vi "Main.vi"(11 "Module Admin":refnum<class "Delacor_lib_QMH_Module Admin.lvclass">) -> ()   [LabVIEW 2020, in "Main.lvlib"]
doc: "This template is based off of the Queued Message Handler design pattern and the Queued Message Handler project template that ships with LabVIEW.\n\nThe main difference is that the queue is private to this module and communication between modules is performed via Broadcast and Request events.\n\nRequest events are wrapped in public API methods and are handled in the Event Handling Loop (EHL) of this VI. Any module can register for Broadcast events sent by this module. The EHL generates messages based on user interface actions.\n\nThe Message Handling Loop (MHL) processes messages generated by the EHL, or by other messages. The messages are string values, so new messages can be added easily to the Message Cases case structure in the MHL. Each message cluster can also provide an optional value for Message Data, which is a variant that can be converted to whatever message-specific data is required.\n_____\nBased on Delacor QMH Project Template 5.0.0.82."
uses:
  Main.lvlib
  <vilib>/Delacor/Delacor QMH/Libraries/Module Admin_class/Delacor_lib_QMH_Module Admin.lvclass
  Module Data--cluster.ctl
  <vilib>/Delacor/Delacor QMH/Libraries/Message Queue_class/Delacor_lib_QMH_Message Queue.lvclass/Delacor_lib_QMH_Message Queue.ctl
  <vilib>/event_ctls.llb/eventvkey.ctl
  Stop Argument--cluster.ctl
  <vilib>/Delacor/Delacor QMH/Libraries/Module Admin_class/Delacor_lib_QMH_Module Admin.lvclass/Delacor_lib_QMH_Module Admin.ctl
  <vilib>/event_ctls.llb/usereventprio.ctl
  <vilib>/Delacor/Delacor QMH/Libraries/Message Queue_class/Delacor_lib_QMH_Enqueue Message (Single).vi
  <vilib>/Delacor/Delacor QMH/Libraries/Module Admin_class/Delacor_lib_QMH_Get External Launch.vi
  <vilib>/Utility/error.llb/Error Cluster From Error Code.vi
  <vilib>/ErrorRing/Error Ring.xnode
  <vilib>/Delacor/Delacor QMH/Libraries/Message Queue_class/Delacor_lib_QMH_Message Queue.lvclass
  History/History.lvlib
  Fallas/Fallas.lvlib
  Pruebas/Pruebas.lvlib
  Graficas/Graficas.lvlib
panel:
  out "stop?":bool
  out "date/time string":string
  out "Enum Param":enum16{"None", "Corriente", "SOC", "Temp"}(ring)=enum."Temp"
  in  "Salir":bool
  in  "Historial":bool
  in  "Pruebas":bool
  in  "Fallas":bool
  in  "Pagina Principal":bool
  in  "OK SOC":bool
  in  "SOC de Batería":dbl min=0.0 max=340.0 step=10.0 format="%#_g %"
  out "Bus DC Encendido":bool
  in  "Ok Temperatura":bool
  in  "Temperatura de Batería":dbl min=0.0 max=340.0 step=10.0 format="%#_g °C"
  in  "Ok Propulsion":bool
  in  "Corriente de Propulsión":dbl min=0.0 max=340.0 step=10.0 format="%#_g A"
  in  "Modo Propulsion":bool
  in  "Conexion a Linea de Carga":bool
  in  "Encender Generador":bool
  out "error out":errorcluster
  out "Status":string
  # "Operación del Sistema"
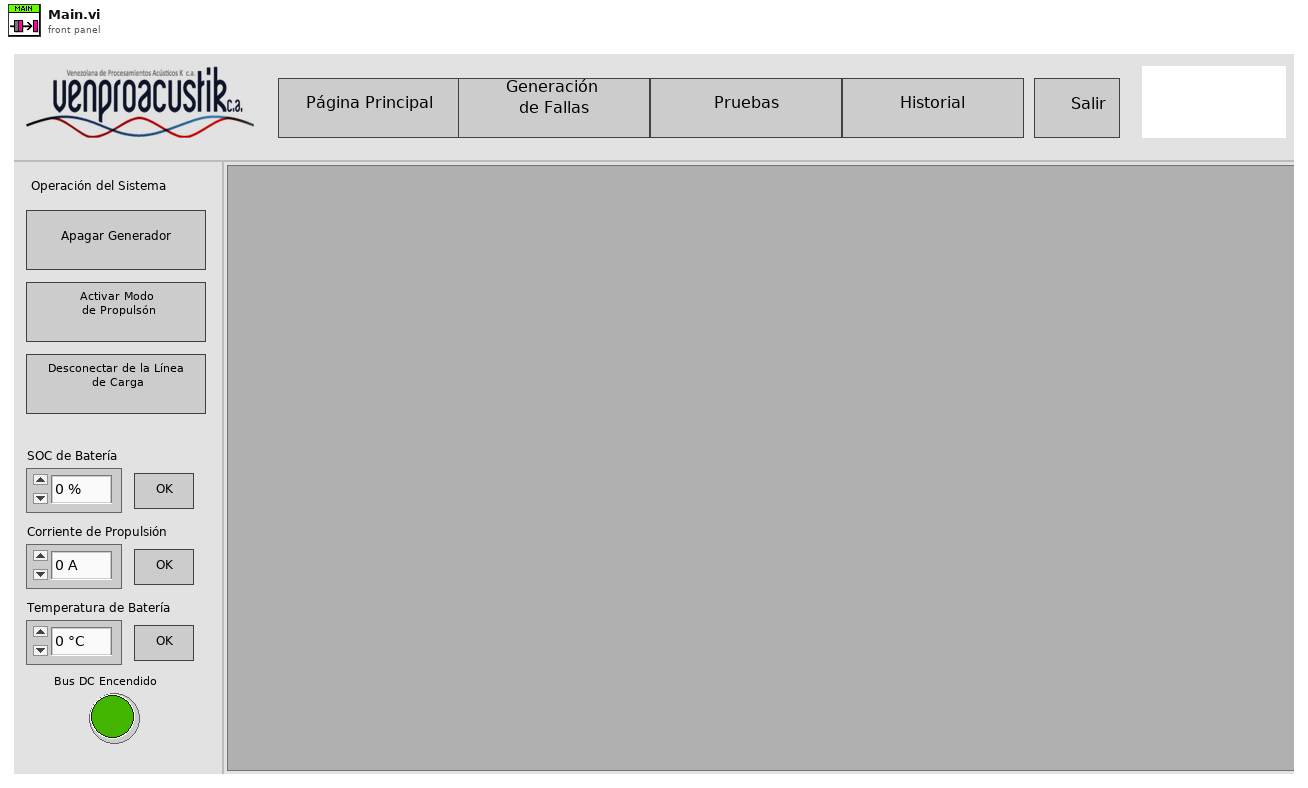
[diagram p1: front panel]
types:
  T1 = typedef "Main.lvlib/Request Events--cluster.ctl" = cluster{"Stop Module":refnum<user-event>, "Show Panel":refnum<user-event>, "Hide Panel":refnum<user-event>, "Get Module Execution Status":refnum<user-event>, "Show Diagram":refnum<user-event>}
  T2 = typedef "History.lvlib/Broadcast Events--cluster.ctl" = cluster{"Module Did Init":refnum<user-event>, "Status Updated":refnum<user-event>, "Error Reported":refnum<user-event>, "Module Did Stop":refnum<user-event>, "Update Module Execution Status":refnum<user-event>}
  T3 = typedef "Fallas.lvlib/Broadcast Events--cluster.ctl" = cluster{"Module Did Init":refnum<user-event>, "Status Updated":refnum<user-event>, "Error Reported":refnum<user-event>, "Module Did Stop":refnum<user-event>, "Update Module Execution Status":refnum<user-event>}
  T4 = typedef "Pruebas.lvlib/Broadcast Events--cluster.ctl" = cluster{"Module Did Init":refnum<user-event>, "Status Updated":refnum<user-event>, "Error Reported":refnum<user-event>, "Module Did Stop":refnum<user-event>, "Update Module Execution Status":refnum<user-event>, "Controles de relés de prueba actualizados":refnum<user-event>, "Valor de Medicion de Prueba Enviado":refnum<user-event>, "Valor de Modulacion Debugging Enviado":refnum<user-event>}
  T5 = typedef "Graficas.lvlib/Broadcast Events--cluster.ctl" = cluster{"Module Did Init":refnum<user-event>, "Status Updated":refnum<user-event>, "Error Reported":refnum<user-event>, "Module Did Stop":refnum<user-event>, "Update Module Execution Status":refnum<user-event>}
  T6 = typedef "Main.lvlib/Module Data--cluster.ctl" = cluster{"Status":string}
  T7 = typedef "eventvkey.ctl" = enum16{"ASCII", "Enter", "Return", "Shift", "Ctrl", "Alt", "Cmd", "Opt", "Caps", "NumLock", "Clear", "Break", "Up", "Down", "Left", "Right", "Insert", "Delete", "Home", "End", "PageUp", "PageDown", "Escape", "Help", "Pause", "ScrollLock", "F1", "F2", "F3", "F4", "F5", "F6", "F7", "F8", "F9", "F10", "F11", "F12", "F13", "F14", "F15", "F16", "F17", "F18", "F19", "F20", "F21", "F22", "F23", "F24", "Play", "VolumeUp", "VolumeDown", "Mute", "Two Byte Char"}
  T8 = typedef "Main.lvlib/Stop Argument--cluster.ctl" = cluster{"Origin":string, "Exit via Stop Module Req?":bool, "Wait for Module to stop?":bool}
  T9 = enum32{"invalid lock state", "Not Locked", "Locked (No Password)", "Password-protected"}
  T10 = typedef "usereventprio.ctl" = enum32{"high priority", "normal priority"}
  T11 = enum32{"Invalid", "Standard", "Closed", "Hidden", "Minimized", "Maximized"}
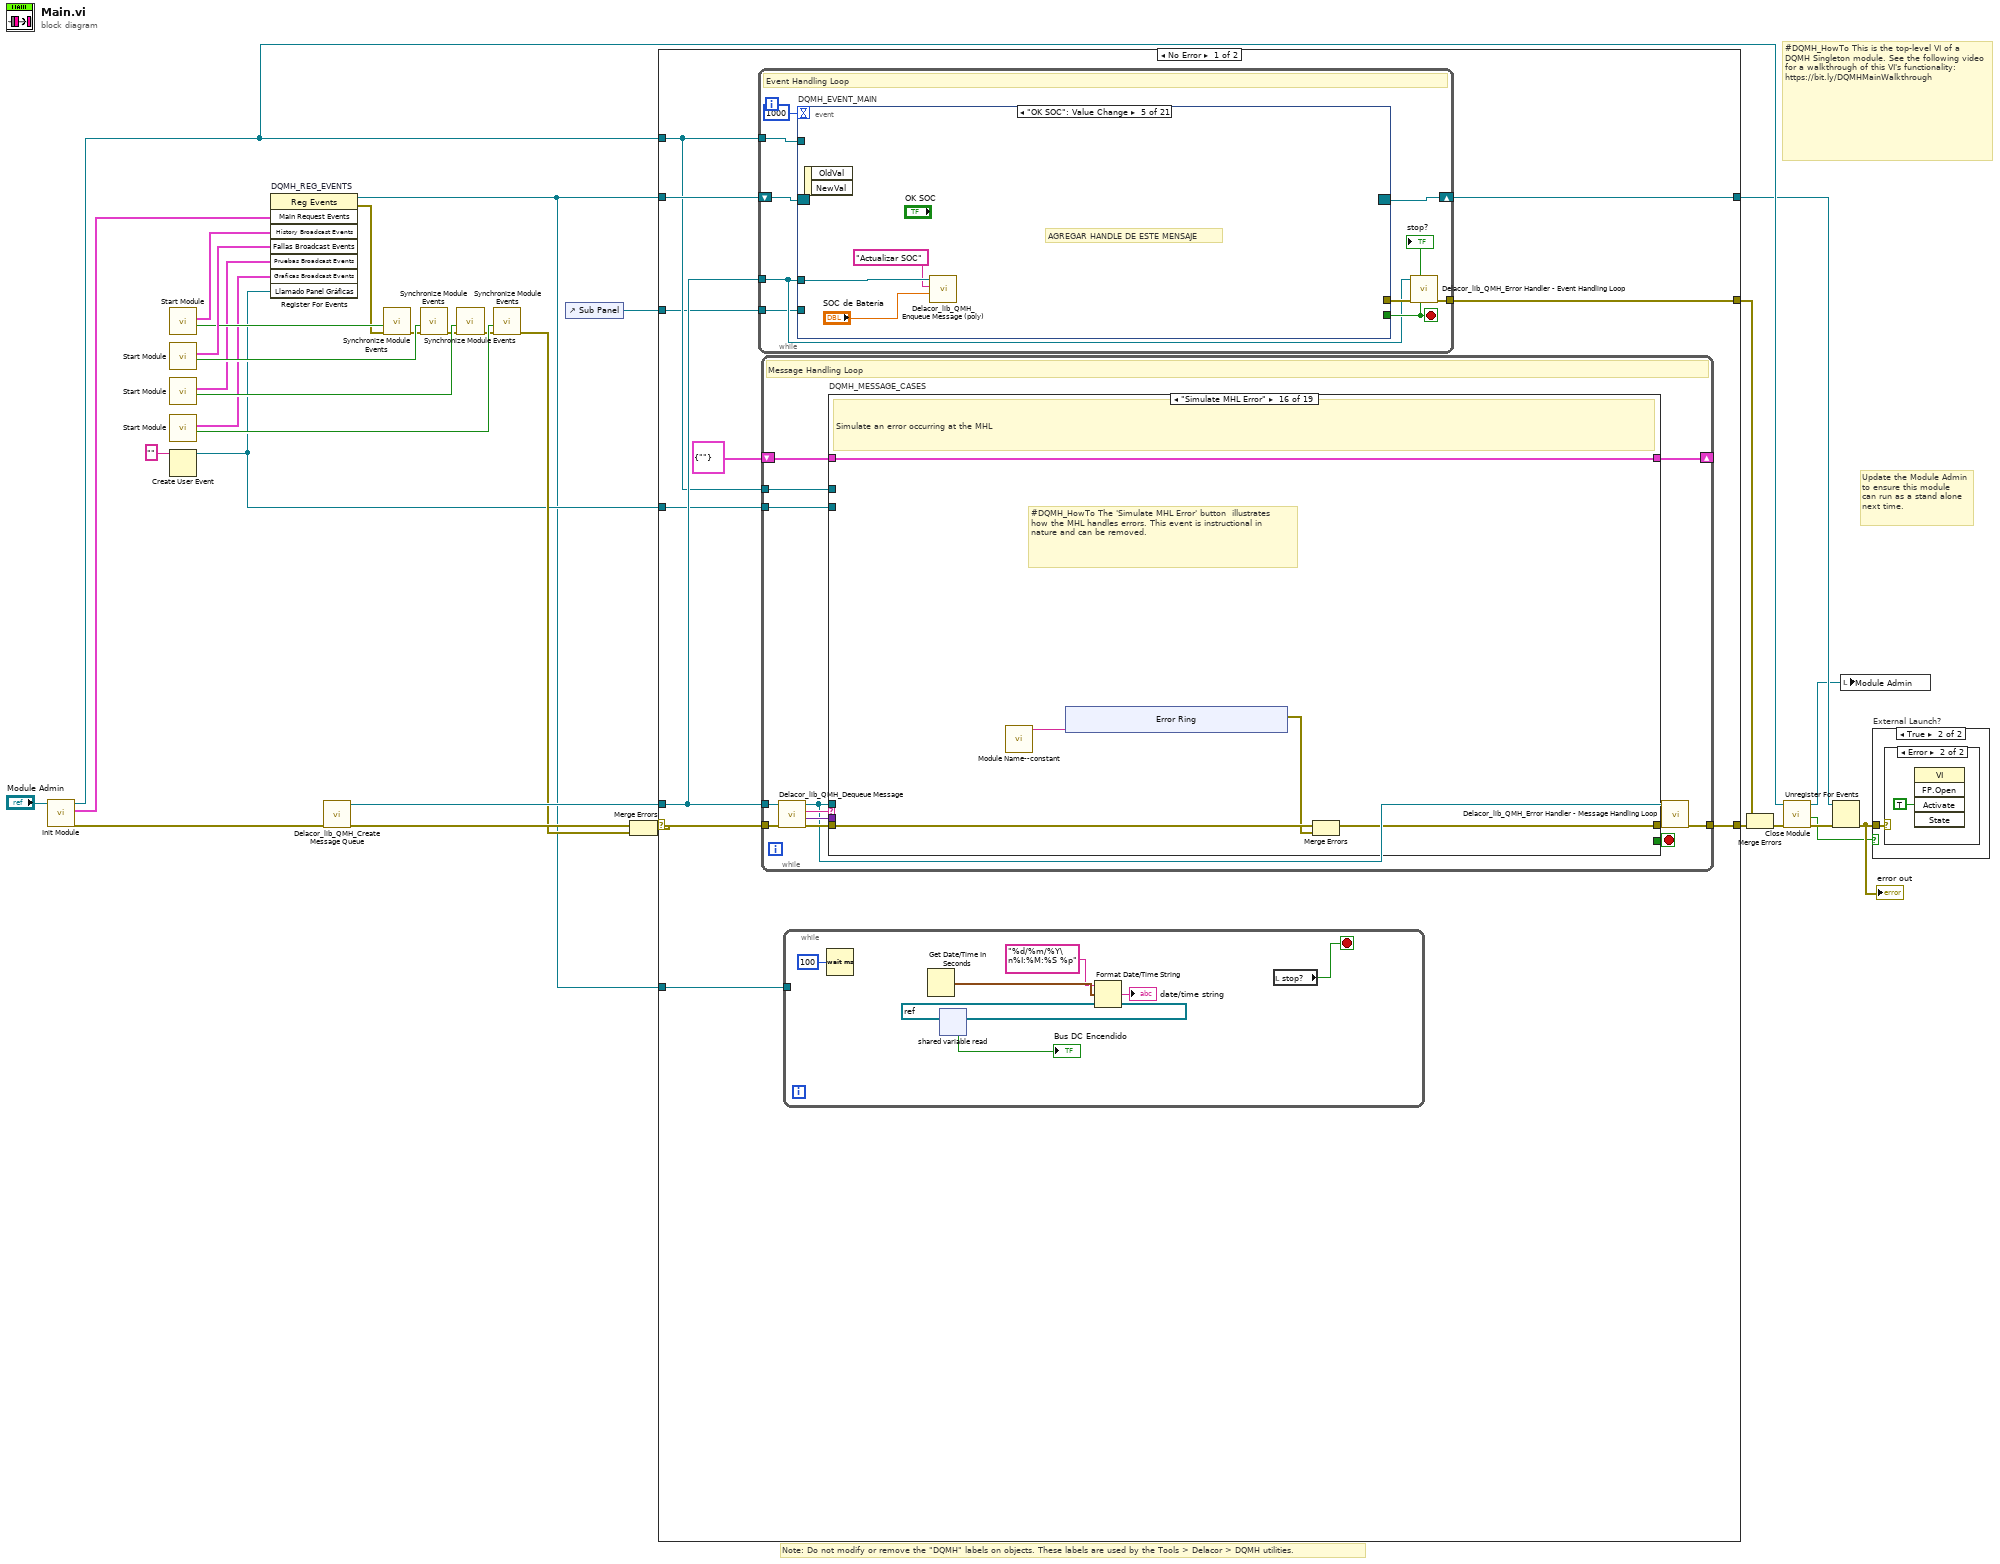
[diagram p0: block diagram]
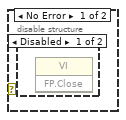
[diagram p3: hidden frame]
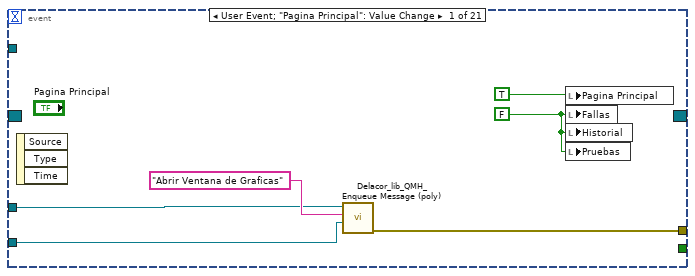
[diagram p5: hidden frame]
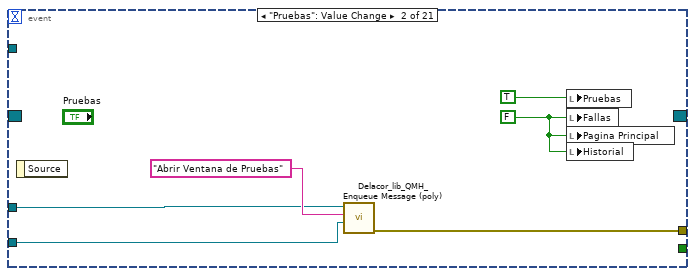
[diagram p6: hidden frame]
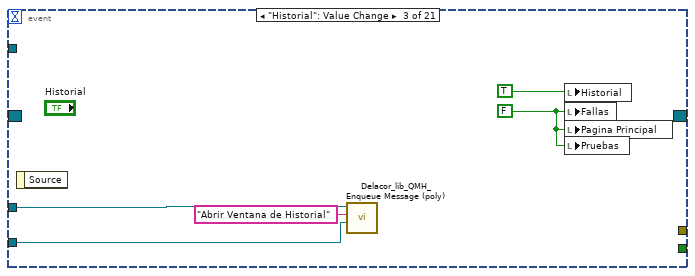
[diagram p7: hidden frame]
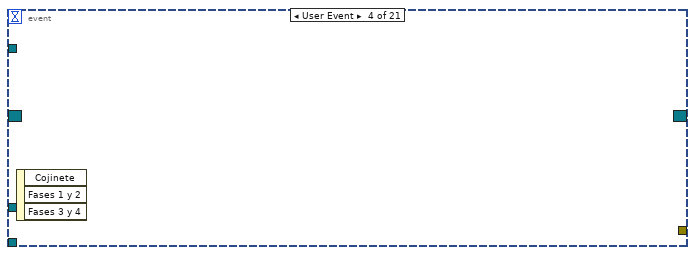
[diagram p8: hidden frame]
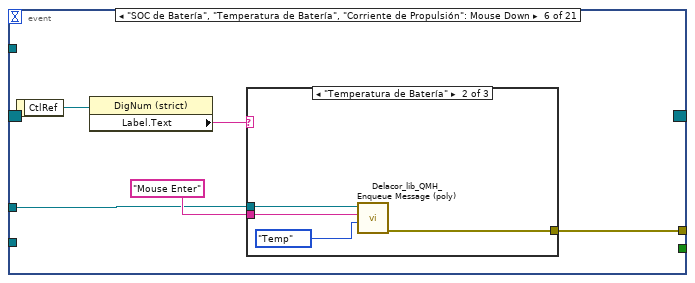
[diagram p9: hidden frame]
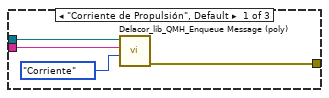
[diagram p10: hidden frame]
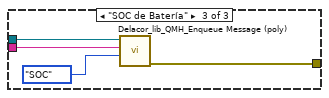
[diagram p11: hidden frame]
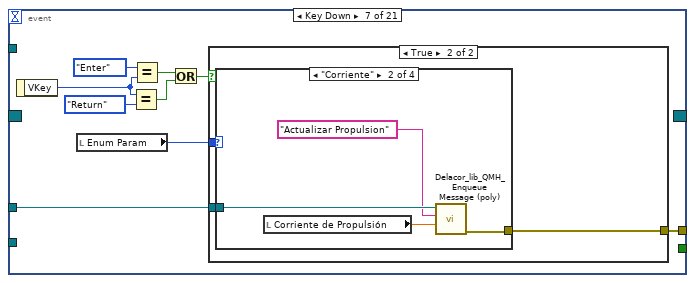
[diagram p12: hidden frame]
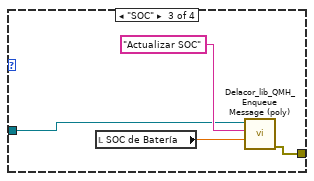
[diagram p15: hidden frame]
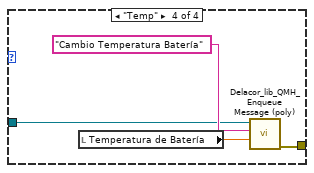
[diagram p16: hidden frame]
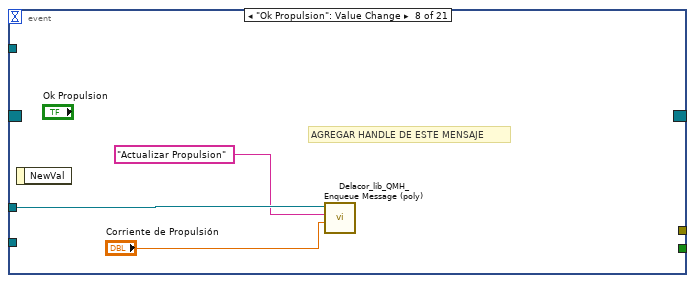
[diagram p17: hidden frame]
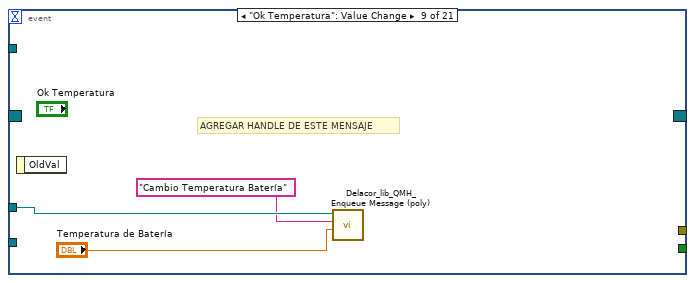
[diagram p18: hidden frame]
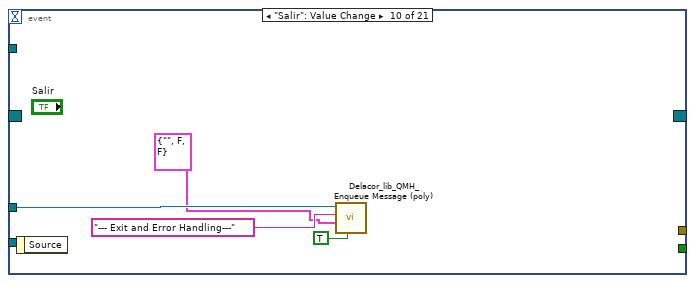
[diagram p19: hidden frame]
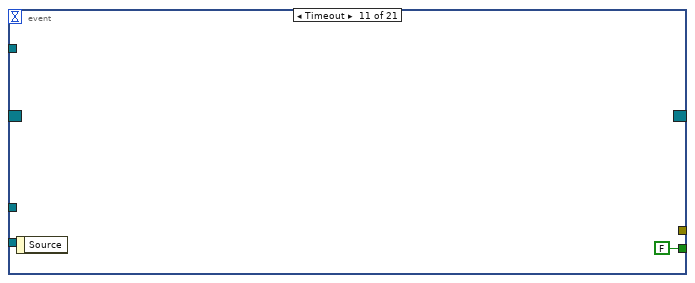
[diagram p20: hidden frame]
diagram:
  # "#DQMH_HowTo This is the top-level VI of a DQMH Singleton module. See the following video for a walkthrough of this VI's functionality: https://bit.ly/DQMHMainWalkthrough"
  # "Note: Do not modify or remove the \"DQMH\" labels on objects. These labels are used by the Tools > Delacor > DQMH utilities."
  # "Update the Module Admin to ensure this module can run as a stand alone next time."
  n1 = call "Init Module.vi"("Singleton Module Admin in"="Module Admin") -> ("error out"=w31:errorcluster, "Main Request Events"=w22:T1, "Singleton Module Admin out"=w24:refnum<class "Delacor_lib_QMH_Module Admin.lvclass">)  [unwired: 8 in]
  n2 = call "Start Module.vi"() -> ("Wait for Event Sync?"=w15:bool, "History Broadcast Events"=w17:T2)  [unwired: 8 in, 2 out]
  n3 = call "Start Module.vi"() -> ("Wait for Event Sync?"=w14:bool, "Fallas Broadcast Events"=w16:T3)  [unwired: 7 in, 3 out]
  n4 = call "Start Module.vi"() -> ("Wait for Event Sync?"=w11:bool, "Pruebas Broadcast Events"=w12:T4)  [unwired: 8 in, 2 out]
  n5 = call "Start Module.vi"() -> ("Wait for Event Sync?"=w9:bool, "Graficas Broadcast Events"=w10:T5)  [unwired: 8 in, 2 out]
  n6 = Create User Event(user event datatype="" ("Llamado Panel Gráficas")) -> (user event=w2:refnum<user-event>)  [unwired: 1 in, 1 out]
  n7 = register-events "DQMH_REG_EVENTS"(w22, w17, w16, w12, w10, w2) -> (reference out=w1:refnum<event-registration>, error out=w8:errorcluster)  [unwired: 2 in]
  n8 = call <vilib>:"Delacor_lib_QMH_Create Message Queue.vi"("error in (no error)"=w31) -> ("error out"=w26:errorcluster, "Message Queue"=w21:refnum<class "Delacor_lib_QMH_Message Queue.lvclass">)  [unwired: 9 in]
  n9 = call "Synchronize Module Events.vi"("error in (no error)"=w8, "Wait for Event Sync?"=w15) -> ("error out"=w7:errorcluster)  [unwired: 9 in]
  n10 = call "Synchronize Module Events.vi"("error in (no error)"=w7, "Wait for Event Sync?"=w14) -> ("error out"=w6:errorcluster)  [unwired: 9 in]
  n11 = call "Synchronize Module Events.vi"("error in (no error)"=w6, "Wait for Event Sync?"=w11) -> ("error out"=w5:errorcluster)  [unwired: 9 in]
  n12 = call "Synchronize Module Events.vi"("error in (no error)"=w5, "Wait for Event Sync?"=w9) -> ("error out"=w4:errorcluster)  [unwired: 9 in]
  n13 = control-ref of="Sub Panel"() -> (w13:refnum<vi>)
  n14 = Merge Errors(w26, w4) -> (w25:errorcluster)
  n15 = case shown="No Error" w25 {
    selector: w25 -> [w41 w408]
    tunnel: [w43 w407] -> w32
    tunnel: [w40 w413] -> w23
    tunnel: w1 -> [w38 w413]
    tunnel: w21 -> [w37 w406]
    tunnel: [w42 _] -> w29
    tunnel: w24 -> [w36 w409]
    tunnel: w13 -> [w35 _]
    tunnel: w2 -> [w34 _]
    tunnel: w1 -> [w33 _]
    frame No Error {
      n16 = while {
        tunnel: w37 -> [w53]
        shift-right: [w56] -> w40
        shift-left: w38 -> [w57]
        tunnel: [w58] -> w42
        tunnel: w36 -> [w54]
        tunnel: w35 -> [w52]
        stop <- w55 stop-if-true
        # "Event Handling Loop"
        n17 = event "DQMH_EVENT_MAIN" shown="[4] \"OK SOC\": Value Change" {
          selector: w57 -> [_ _ _ _ _ _ _ _ _ _ _ _ _ _ _ _ _ _ _ _ _]
          dyn-events: [_ _ _ _ _ _ _ _ _ _ _ _ _ _ _ _ _ _ _ _ _] -> w56
          timeout: 1000 -> [_ _ _ _ _ _ _ _ _ _ _ _ _ _ _ _ _ _ _ _ _]
          tunnel: [_ _ _ _ _ _ _ _ _ _ FALSE ("Discard?") _ _ _ _ _ TRUE ("Discard?") _ _ _ _] -> w55
          tunnel: w53 -> [w62 w66 w76 _ w79 w80 w98 w123 w126 w129 _ w136 _ _ _ _ w160 w168 w171 w175 w179]
          tunnel: [w61 w67 _ _ _ w82 w97 _ _ _ _ w132 _ _ w143 _ w163 w165 w170 w174 w181] -> w59
          tunnel: w54 -> [_ _ _ _ _ _ _ _ _ _ _ _ _ _ _ _ _ _ _ _ w178]
          tunnel: w52 -> [w60 w68 w72 _ _ _ _ _ _ _ _ w133 _ _ _ _ _ _ _ _ _]
          event User Event; "Pagina Principal": Value Change {
            w65 = FALSE ("Fallas")
            n18 = event-data() -> ()  [unwired: 1 in, 3 out]
            n19 = call-poly <vilib>:"Delacor_lib_QMH_Enqueue Message (poly).vi"("Message Data"=w60, "Message"="Abrir Ventana de Graficas", "Message Queue in"=w62) -> ("error out"=w61:errorcluster)  [unwired: 7 in, 1 out]
            n20 = local write "Pagina Principal"(TRUE ("Fallas")) -> ()
            n21 = local write "Fallas"(w65) -> ()
            n22 = local write "Historial"(w65) -> ()
            n23 = local write "Pruebas"(w65) -> ()
          }
          event "Pruebas": Value Change {
            w71 = FALSE ("Fallas")
            n24 = event-data() -> ()  [unwired: 1 in, 1 out]
            n25 = call-poly <vilib>:"Delacor_lib_QMH_Enqueue Message (poly).vi"("Message Data"=w68, "Message"="Abrir Ventana de Pruebas", "Message Queue in"=w66) -> ("error out"=w67:errorcluster)  [unwired: 7 in, 1 out]
            n26 = local write "Pruebas"(TRUE ("Fallas")) -> ()
            n27 = local write "Fallas"(w71) -> ()
            n28 = local write "Pagina Principal"(w71) -> ()
            n29 = local write "Historial"(w71) -> ()
          }
          event "Historial": Value Change {
            w74 = FALSE ("Fallas")
            n30 = event-data() -> ()  [unwired: 1 in, 1 out]
            n31 = call-poly <vilib>:"Delacor_lib_QMH_Enqueue Message (poly).vi"("Message Data"=w72, "Message"="Abrir Ventana de Historial", "Message Queue in"=w76) -> ()  [unwired: 7 in, 2 out]
            n32 = local write "Historial"(TRUE ("Fallas")) -> ()
            n33 = local write "Fallas"(w74) -> ()
            n34 = local write "Pagina Principal"(w74) -> ()
            n35 = local write "Pruebas"(w74) -> ()
          }
          event User Event {
            n36 = event-data() -> ()  [unwired: 1 in, 3 out]
          }
          event "OK SOC": Value Change {
            # "AGREGAR HANDLE DE ESTE MENSAJE"
            n37 = event-data() -> ()  [unwired: 1 in, 2 out]
            n38 = call-poly <vilib>:"Delacor_lib_QMH_Enqueue Message (poly).vi"("Message Data"="SOC de Batería", "Message"="Actualizar SOC", "Message Queue in"=w79) -> ()  [unwired: 7 in, 2 out]
          }
          event "SOC de Batería", "Temperatura de Batería", "Corriente de Propulsión": Mouse Down {
            n39 = event-data() -> ("CtlRef"=w84:refnum<vi>)  [unwired: 1 in]
            n40 = property class="DigNum (strict)"(reference=w84) -> ("Label.Text"=w83:string)  [unwired: 1 in, 2 out]
            n41 = case shown="\"Temperatura de Batería\"" w83 {
              tunnel: w80 -> [w88 w92 w96]
              tunnel: [w87 w91 w95] -> w82
              tunnel: "Mouse Enter" ("Message") -> [w85 w90 w93]
              frame "Corriente de Propulsión", Default {
                n42 = call-poly <vilib>:"Delacor_lib_QMH_Enqueue Message (poly).vi"("Message Data"=enum16{"None", "Corriente", "SOC", "Temp"}."Corriente", "Message"=w85, "Message Queue in"=w88) -> ("error out"=w87:errorcluster)  [unwired: 7 in, 1 out]
              }
              frame "Temperatura de Batería" {
                n43 = call-poly <vilib>:"Delacor_lib_QMH_Enqueue Message (poly).vi"("Message Data"=enum16{"None", "Corriente", "SOC", "Temp"}."Temp", "Message"=w90, "Message Queue in"=w92) -> ("error out"=w91:errorcluster)  [unwired: 7 in, 1 out]
              }
              frame "SOC de Batería" {
                n44 = call-poly <vilib>:"Delacor_lib_QMH_Enqueue Message (poly).vi"("Message Data"=enum16{"None", "Corriente", "SOC", "Temp"}."SOC", "Message"=w93, "Message Queue in"=w96) -> ("error out"=w95:errorcluster)  [unwired: 7 in, 1 out]
              }
            }
          }
          event Key Down {
            n45 = event-data() -> ("VKey"=w104:T7)  [unwired: 1 in]
            n46 = local read "Enum Param"() -> (w99:enum16{"None", "Corriente", "SOC", "Temp"})
            n47 = Equal?(x=w104, y=eventvkey."Return" ("VKey 2")) -> (x = y?=w101:bool)
            n48 = Equal?(x=eventvkey."Enter" ("VKey 2"), y=w104) -> (x = y?=w102:bool)
            n49 = Or(x=w102, y=w101) -> (x .or. y?=w100:bool)
            n50 = case shown="True" w100 {
              tunnel: w99 -> [_ w108]
              tunnel: w98 -> [_ w107]
              tunnel: [_ w106] -> w97
              frame False {
              }
              frame True {
                n51 = case shown="\"Corriente\"" w108 {
                  tunnel: w107 -> [_ w112 w114 w118]
                  tunnel: [_ w111 w113 w117] -> w106
                  frame "None", Default {
                  }
                  frame "Corriente" {
                    n52 = local read "Corriente de Propulsión"() -> (w109:dbl)
                    n53 = call-poly <vilib>:"Delacor_lib_QMH_Enqueue Message (poly).vi"("Message Data"=w109, "Message"="Actualizar Propulsion", "Message Queue in"=w112) -> ("error out"=w111:errorcluster)  [unwired: 7 in, 1 out]
                  }
                  frame "SOC" {
                    n54 = local read "SOC de Batería"() -> (w116:dbl)
                    n55 = call-poly <vilib>:"Delacor_lib_QMH_Enqueue Message (poly).vi"("Message Data"=w116, "Message"="Actualizar SOC", "Message Queue in"=w114) -> ("error out"=w113:errorcluster)  [unwired: 7 in, 1 out]
                  }
                  frame "Temp" {
                    n56 = local read "Temperatura de Batería"() -> (w120:dbl)
                    n57 = call-poly <vilib>:"Delacor_lib_QMH_Enqueue Message (poly).vi"("Message Data"=w120, "Message"="Cambio Temperatura Batería", "Message Queue in"=w118) -> ("error out"=w117:errorcluster)  [unwired: 7 in, 1 out]
                  }
                }
              }
            }
          }
          event "Ok Propulsion": Value Change {
            # "AGREGAR HANDLE DE ESTE MENSAJE"
            n58 = event-data() -> ()  [unwired: 1 in, 1 out]
            n59 = call-poly <vilib>:"Delacor_lib_QMH_Enqueue Message (poly).vi"("Message Data"="Corriente de Propulsión", "Message"="Actualizar Propulsion", "Message Queue in"=w123) -> ()  [unwired: 7 in, 2 out]
          }
          event "Ok Temperatura": Value Change {
            # "AGREGAR HANDLE DE ESTE MENSAJE"
            n60 = event-data() -> ()  [unwired: 1 in, 1 out]
            n61 = call-poly <vilib>:"Delacor_lib_QMH_Enqueue Message (poly).vi"("Message Data"="Temperatura de Batería", "Message"="Cambio Temperatura Batería", "Message Queue in"=w126) -> ()  [unwired: 7 in, 2 out]
          }
          event "Salir": Value Change {
            n62 = event-data() -> ()  [unwired: 1 in, 1 out]
            n63 = call-poly <vilib>:"Delacor_lib_QMH_Enqueue Message (poly).vi"("Priority Message? (F)"=TRUE, "Message Data"=T8 {"Origin"="", "Exit via Stop Module Req?"=FALSE, "Wait for Module to stop?"=FALSE} ("Stop Argument"), "Message"="--- Exit and Error Handling---", "Message Queue in"=w129) -> ()  [unwired: 6 in, 2 out]
          }
          event Timeout {
            n64 = event-data() -> ()  [unwired: 1 in, 1 out]
          }
          event "Fallas": Value Change {
            w134 = FALSE ("Fallas")
            n65 = event-data() -> ()  [unwired: 1 in, 1 out]
            n66 = call-poly <vilib>:"Delacor_lib_QMH_Enqueue Message (poly).vi"("Message Data"=w133, "Message"="Abrir Ventana de Fallas", "Message Queue in"=w136) -> ("error out"=w132:errorcluster)  [unwired: 7 in, 1 out]
            n67 = local write "Fallas"(TRUE ("Fallas")) -> ()
            n68 = local write "Historial"(w134) -> ()
            n69 = local write "Pagina Principal"(w134) -> ()
            n70 = local write "Pruebas"(w134) -> ()
          }
          event User Event {
            # "Show the panel of this VI, and send a status updated message to let listeners know."
            # "Another Module called the \"Show Panel\" API Method."
            n71 = event-data() -> ()  [unwired: 1 in, 1 out]
            n72 = control-ref of="This VI"() -> (w139:refnum<vi>)
            n73 = call "Open VI Panel.vi"("VI"=w139) -> ()  [unwired: 10 in, 1 out]
            n74 = call "Status Updated.vi"("Status"="Panel shown." ("format string")) -> ()  [unwired: 10 in, 1 out]
          }
          event User Event {
            # "Hide the panel of this VI, and send a status updated message to let listeners know."
            # "Another Module called the \"Hide Panel\" API Method."
            n75 = event-data() -> ()  [unwired: 1 in, 1 out]
            n76 = control-ref of="This VI"() -> (w141:refnum<vi>)
            n77 = call "Hide VI Panel.vi"("VI"=w141) -> ()  [unwired: 10 in, 1 out]
            n78 = call "Status Updated.vi"("Status"="Panel hidden." ("format string")) -> ()  [unwired: 10 in, 1 out]
          }
          event User Event {
            # "Another Module called the \"Get Module Execution Status\" API Method."
            n79 = event-data() -> ()  [unwired: 1 in, 1 out]
            n80 = call "Update Module Execution Status.vi"("Running?"=TRUE) -> ("error out"=w143:errorcluster)  [unwired: 10 in]
          }
          event User Event {
            # "Another Module called the \"Show Diagram\" API Method. This event is used for debugging."
            n81 = event-data() -> ()  [unwired: 1 in, 1 out]
            n82 = disable-structure shown="Default" {
              frame condition #0 (active) {
                # "functionality not available in exe"
                n83 = invoke class="VI" method="Lock State.Get"() -> (error out=w149:errorcluster, "Get Lock State"=w148:T9, "pwd in cache"=w145:bool)  [unwired: 4 in, 1 out]
                n84 = Equal?(x=T9."Password-protected", y=w148) -> (x = y?=w146:bool)
                n85 = Compound Arithmetic op=AND(w146, invert w145) -> (w144:bool)
                n86 = case shown="False" w144 {
                  tunnel: w149 -> [w152 _]
                  frame False {
                    n87 = property class="VI"(error in=w152, "BDWin.Open"=TRUE ("Block Diagram Window:Open")) -> ()  [unwired: 1 in, 2 out]
                    n88 = call "Status Updated.vi"("Status"="Block Diagram shown." ("format string")) -> ()  [unwired: 10 in, 1 out]
                  }
                  frame True {
                    # "Password-protected VI, and the password is not in the cache. Do not show the diagram."
                  }
                }
              }
              frame condition #1 {
              }
            }
          }
          event User Event {
            # "The Stop Module Event can get fired from the Exit message in the MHL. The queue gets destroyed in that case. If the queue no longer exists, the Enqueue Exit as a priority message will return error 1. It is safe to ignore, because the module is already exiting."
            # "Another Module called the \"Stop Module\" API Method  or the Message Handling Loop below."
            n89 = event-data() -> ("Origin"=w159:string, "Exit via Stop Module Req?"=w155:bool, "Wait for Module to stop?"=w154:bool)  [unwired: 1 in]
            n90 = local write "Status"(w159) -> ()
            n91 = Bundle By Name(cluster=T8 {"Origin"="", "Exit via Stop Module Req?"=FALSE, "Wait for Module to stop?"=FALSE} ("Stop Argument"), "Exit via Stop Module Req?"=w155, "Wait for Module to stop?"=w154) -> (w153:T8)
            n92 = call-poly <vilib>:"Delacor_lib_QMH_Enqueue Message (poly).vi"("Priority Message? (F)"=TRUE, "Message Data"=w153, "Message"="Exit", "Message Queue in"=w160) -> ("error out"=w164:errorcluster)  [unwired: 6 in, 1 out]
            n93 = call <vilib>:"Clear Errors.vi"("error in (no error)"=w164, "specific error code to clear (0: all)"=1) -> ("error out"=w163:errorcluster)  [unwired: 4 in, 1 out]
          }
          event "Encender Generador": Value Change {
            n94 = event-data() -> ()  [unwired: 1 in, 1 out]
            n95 = call-poly <vilib>:"Delacor_lib_QMH_Enqueue Message (poly).vi"("Message Data"="Encender Generador", "Message"="Boton Encender Generador Presionado", "Message Queue in"=w168) -> ("error out"=w165:errorcluster)  [unwired: 7 in, 1 out]
          }
          event "Conexion a Linea de Carga": Value Change {
            n96 = event-data() -> ()  [unwired: 1 in, 1 out]
            n97 = call-poly <vilib>:"Delacor_lib_QMH_Enqueue Message (poly).vi"("Message Data"="Conexion a Linea de Carga", "Message"="Boton Conexión a Linea de Caga Presionado", "Message Queue in"=w171) -> ("error out"=w170:errorcluster)  [unwired: 7 in, 1 out]
          }
          event "Modo Propulsion": Value Change {
            n98 = event-data() -> ()  [unwired: 1 in, 1 out]
            n99 = call-poly <vilib>:"Delacor_lib_QMH_Enqueue Message (poly).vi"("Message Data"="Modo Propulsion", "Message"="Boton Modo Propulsion Presionado", "Message Queue in"=w175) -> ("error out"=w174:errorcluster)  [unwired: 7 in, 1 out]
          }
          event Panel Close? {
            w180 = TRUE  # Discard the event, the MHL is responsible for closing and stopping this VI.
            # "Hide the panel or send the 'Exit' message if the user clicks the 'X' on the module main VI panel."
            n100 = event-data() -> ()  [unwired: 1 in, 1 out]
            n101 = property class="Module Admin"(reference=w178) -> ("Accessors:External Launch"=w177:bool)  [unwired: 1 in, 2 out]
            n102 = case shown="True" w177 {
              tunnel: w179 -> [_ w185]
              tunnel: [_ w186] -> w181
              frame True {
                # "If externally launched, clicking the 'X' hides the panel, but doesn't close it."
                n103 = control-ref of="This VI"() -> (w182:refnum<vi>)
                n104 = call "Hide VI Panel.vi"("VI"=w182) -> ()  [unwired: 10 in, 1 out]
              }
              frame False {
                # "If run as a stand-alone VI, clicking the panel 'X' stops the VI."
                n105 = call-poly <vilib>:"Delacor_lib_QMH_Enqueue Message (poly).vi"("Priority Message? (F)"=TRUE, "Message"="Exit", "Message Queue in"=w185) -> ("error out"=w186:errorcluster)  [unwired: 7 in, 1 out]
              }
            }
            n106 = event-data("Discard?"=w180) -> ()  [unwired: 1 in, 1 out]
          }
        }
        "stop?" <- w55
        n107 = call-dynamic "Delacor_lib_QMH_Error Handler - Event Handling Loop.vi"("error in (no error)"=w59, "Message Queue in"=w53) -> ("dup error in"=w58:errorcluster)  [unwired: 8 in, 1 out]
      }
      n108 = while {
        tunnel: w37 -> [w190]
        shift-right: [w194] -> _
        shift-left: T6 {"Status"=""} ("Data Cluster") -> [w195]
        tunnel: w41 -> [w198]
        tunnel: [w196] -> w43
        tunnel: w36 -> [w188]
        tunnel: w34 -> [w187]
        stop <- w193 stop-if-true
        # "Message Handling Loop"
        n109 = call-dynamic "Delacor_lib_QMH_Dequeue Message.vi"("error in (no error)"=w198, "Message Queue in"=w190) -> ("error out"=w197:errorcluster, "Message Data"=w191:variant, "Message"=w192:string, "Message Queue out"=w189:refnum<class "Delacor_lib_QMH_Message Queue.lvclass">)  [unwired: 6 in]
        n110 = case "DQMH_MESSAGE_CASES" shown="\"Simulate MHL Error\"" w192 {
          selector: w192 -> [_ _ _ _ _ _ _ _ _ _ _ _ _ _ _ _ _ _ w393]
          tunnel: w189 -> [_ _ _ _ _ _ _ _ _ _ _ _ _ _ w346 _ w363 w385 _]
          tunnel: w197 -> [w227 w231 w234 w241 w251 w260 w268 w282 w293 w302 w318 w326 w328 w341 _ w352 w370 w391 w395]
          tunnel: [w201 w231 w233 w243 w253 w262 w270 w284 w291 w304 w317 w325 w327 w340 w342 w351 w366 w388 w396] -> w199
          tunnel: w195 -> [w217 w230 w232 w242 w252 w261 w269 w283 w296 w303 w316 w324 w333 w339 w347 w349 w365 w384 w394]
          tunnel: [w216 w230 w232 w242 w252 w261 w269 w283 w296 w303 w316 w324 w333 w339 w347 w349 w365 w384 w394] -> w194
          tunnel: [_ _ _ _ _ _ _ _ _ _ _ _ _ _ _ _ _ w383 _] -> w193
          tunnel: w191 -> [_ _ _ w238 w248 w257 w265 w279 w294 w299 w314 w322 w331 w338 _ _ w364 w382 _]
          tunnel: w188 -> [w218 _ _ _ _ _ _ _ _ _ _ _ _ _ _ _ w362 w377 _]
          tunnel: w187 -> [w211 _ _ _ _ _ _ _ _ _ _ _ _ _ _ _ _ _ _]
          frame "Initialize" {
            w203 = FALSE ("Encender Generador")
            w207 = 0.0 ("Corriente de Propulsión")
            w212 = "Initial Message" ("Initial Message")
            # "Initialize - Any operation that needs to be done before the module can receive messages. Synchronize Caller Events.vi will inform Start Module.vi that the module has launched and is ready to receive messages. Module Did Init.vi will broadcast that the module initialized."
            n111 = call "Synchronize Caller Events.vi"("error in (no error)"=w227, "Singleton Module Admin in"=w218) -> ("error out"=w226:errorcluster, "Singleton Module Admin out"=w213:refnum<class "Delacor_lib_QMH_Module Admin.lvclass">)  [unwired: 8 in]
            n112 = property class="Module Admin"(reference=w213) -> ("Accessors:External Launch"=w222:bool)  [unwired: 1 in, 2 out]
            n113 = local write "SOC de Batería"(w207) -> ()
            n114 = local write "Corriente de Propulsión"(w207) -> ()
            n115 = local write "Temperatura de Batería"(w207) -> ()
            n116 = property on="Encender Generador" class="Bool (strict)"("BoolText.Text"="Encender Generador" ("Boolean Text.Text")) -> ()  [unwired: 2 in, 2 out]
            n117 = property on="Modo Propulsion" class="Bool (strict)"("BoolText.Text"="Activar Modo\n de Propulsón" ("Boolean Text.Text")) -> ()  [unwired: 2 in, 2 out]
            n118 = property on="Conexion a Linea de Carga" class="Bool (strict)"("BoolText.Text"="Conectar a la Línea \nde Carga" ("Boolean Text.Text")) -> ()  [unwired: 2 in, 2 out]
            n119 = Select(t=T11."Hidden" ("State"), s=w222, f=T11."Standard" ("State")) -> (s? t:f=w219:T11)
            n120 = call "Module Name--constant.vi"() -> ("Module Name"=w225:string)  [unwired: 11 in]
            n121 = call "Generador Encendido-Apagado.vi"("Estatus del Generador"=FALSE) -> ()  [unwired: 10 in, 1 out]
            n122 = property class="VI"("Front Panel.Title"=w225) -> (reference out=w224:refnum<vi>, error out=w229:errorcluster)  [unwired: 2 in]
            n123 = local write "Encender Generador"(w203) -> ()
            n124 = local write "Conexion a Linea de Carga"(w203) -> ()
            n125 = local write "Modo Propulsion"(w203) -> ()
            n126 = call "Module Name--constant.vi"() -> ("Module Name"=w214:string)  [unwired: 11 in]
            n127 = local write "stop?"(FALSE ("Discard?")) -> ()
            n128 = invoke class="VI" method="FP.Open"(reference=w224, error in=w229, "State"=w219) -> (reference out=w223:refnum<vi>, error out=w228:errorcluster)  [unwired: 2 in, 3 out]
            n129 = call "Module Did Init.vi"("error in (no error)"=w226, "Initialized?"=TRUE, "Origin"=w214) -> ("error out"=w202:errorcluster)  [unwired: 8 in]
            n130 = Bundle By Name(cluster=w217, "Status"=w212) -> (w216:T6)
            n131 = invoke class="VI" method="FP.Center"(reference=w223, error in=w228) -> ()  [unwired: 1 in, 3 out]
            n132 = Generate User Event(priority (normal)=usereventprio."high priority", user event=w211, event data cluster="" ("event data"), error in=w202) -> (error out=w201:errorcluster)  [unwired: 1 out]
            "Status" <- w212
          }
          frame "--- Module Specific ---" {
            # "Separator -- The following cases handle messages specific to this Module."
          }
          frame "---Copy This Frame---" {
            # "Duplicate this frame when creating new messages.  Change this comment in the duplicated frame to describe this message."
            n133 = Merge Errors(w234) -> (w233:errorcluster)
          }
          frame "Actualizar SOC" {
            # "Duplicate this frame when creating new messages.  Change this comment in the duplicated frame to describe this message."
            n134 = Variant To Data(error in=w241, type=0.0, Variant=w238) -> (data=w236:dbl, error out=w240:errorcluster)
            n135 = shared-variable-write(refnum<k21> "ni.var.psp://EmuGenV2/VariablesEmuGenV2/SOC Inicial" ("shared variable refnum in"), w236) -> ()  [unwired: 1 in, 2 out]
            n136 = local write "Enum Param"(enum16{"None", "Corriente", "SOC", "Temp"}."None") -> ()
            n137 = Merge Errors(w240) -> (w243:errorcluster)
          }
          frame "Actualizar Propulsion" {
            # "Duplicate this frame when creating new messages.  Change this comment in the duplicated frame to describe this message."
            n138 = Variant To Data(error in=w251, type=0.0, Variant=w248) -> (data=w246:dbl, error out=w250:errorcluster)
            n139 = Negate(x=w246) -> (-x=w245:dbl)
            n140 = Merge Errors(w250) -> (w253:errorcluster)
            n141 = shared-variable-write(refnum<k21> "ni.var.psp://EmuGenV2/VariablesEmuGenV2/Corriente Propulsion" ("shared variable refnum in"), w245) -> ()  [unwired: 1 in, 2 out]
            n142 = local write "Enum Param"(enum16{"None", "Corriente", "SOC", "Temp"}."None") -> ()
          }
          frame "Cambio Temperatura Batería" {
            # "Duplicate this frame when creating new messages.  Change this comment in the duplicated frame to describe this message."
            n143 = Variant To Data(error in=w260, type=0.0, Variant=w257) -> (data=w255:dbl, error out=w259:errorcluster)
            n144 = local write "Enum Param"(enum16{"None", "Corriente", "SOC", "Temp"}."None") -> ()
            n145 = Merge Errors(w259) -> (w262:errorcluster)
            n146 = shared-variable-write(refnum<k21> "ni.var.psp://EmuGenV2/VariablesEmuGenV2/T_Bat_HMI" ("shared variable refnum in"), w255) -> ()  [unwired: 1 in, 2 out]
          }
          frame "Boton Encender Generador Presionado" {
            # "Duplicate this frame when creating new messages.  Change this comment in the duplicated frame to describe this message."
            n147 = Variant To Data(error in=w268, type=FALSE, Variant=w265) -> (data=w264:bool, error out=w267:errorcluster)
            n148 = call "Generador Encendido-Apagado.vi"("Estatus del Generador"=w264) -> ()  [unwired: 10 in, 1 out]
            n149 = case shown="True" w264 {
              selector: w264 -> [w271 w275]
              frame False {
                n150 = call "Agregar evento al historial.vi"("Evento.nombre"="Generador Apagado", "Evento.valor"=w271) -> ()  [unwired: 9 in, 1 out]
                n151 = property on="Encender Generador" class="Bool (strict)"("BoolText.Text"="Encender Generador" ("Boolean Text.Text")) -> ()  [unwired: 2 in, 2 out]
              }
              frame True {
                n152 = call "Agregar evento al historial.vi"("Evento.nombre"="Generador Encendido", "Evento.valor"=w275) -> ()  [unwired: 9 in, 1 out]
                n153 = property on="Encender Generador" class="Bool (strict)"("BoolText.Text"="Apagar Generador" ("Boolean Text.Text")) -> ()  [unwired: 2 in, 2 out]
              }
            }
            n154 = shared-variable-write(refnum<k21> "ni.var.psp://EmuGenV2/VariablesEmuGenV2/ON_OFF" ("shared variable refnum in"), w264) -> ()  [unwired: 1 in, 2 out]
            n155 = Merge Errors(w267) -> (w270:errorcluster)
          }
          frame "Boton Conexión a Linea de Caga Presionado" {
            # "Duplicate this frame when creating new messages.  Change this comment in the duplicated frame to describe this message."
            n156 = Variant To Data(error in=w282, type=FALSE, Variant=w279) -> (data=w278:bool, error out=w281:errorcluster)
            n157 = case shown="False" w278 {
              selector: w278 -> [w286 w290]
              frame False {
                n158 = call "Agregar evento al historial.vi"("Evento.nombre"="Línea de Carga Desconectada", "Evento.valor"=w286) -> ()  [unwired: 9 in, 1 out]
                n159 = property on="Conexion a Linea de Carga" class="Bool (strict)"("BoolText.Text"="Conectar a la Línea \nde Carga" ("Boolean Text.Text")) -> ()  [unwired: 2 in, 2 out]
              }
              frame True {
                n160 = call "Agregar evento al historial.vi"("Evento.nombre"="Línea de Carga Conectada", "Evento.valor"=w290) -> ()  [unwired: 9 in, 1 out]
                n161 = property on="Conexion a Linea de Carga" class="Bool (strict)"("BoolText.Text"="Desconectar de la Línea\n de Carga" ("Boolean Text.Text")) -> ()  [unwired: 2 in, 2 out]
              }
            }
            n162 = Merge Errors(w281) -> (w284:errorcluster)
            n163 = shared-variable-write(refnum<k21> "ni.var.psp://EmuGenV2/VariablesEmuGenV2/Conexion a Linea de Carga" ("shared variable refnum in"), w278) -> ()  [unwired: 1 in, 2 out]
          }
          frame "Mouse Enter" {
            n164 = Variant To Data(error in=w293, type=enum16{"None", "Corriente", "SOC", "Temp"}."Temp", Variant=w294) -> (data=→"Enum Param":enum16{"None", "Corriente", "SOC", "Temp"}, error out=w291:errorcluster)
          }
          frame "Boton Modo Propulsion Presionado" {
            # "Duplicate this frame when creating new messages.  Change this comment in the duplicated frame to describe this message."
            n165 = Variant To Data(error in=w302, type=FALSE, Variant=w299) -> (data=w298:bool, error out=w301:errorcluster)
            n166 = case shown="False" w298 {
              selector: w298 -> [w306 w310]
              frame False {
                n167 = call "Agregar evento al historial.vi"("Evento.nombre"="Modo Propulsión Desactivado", "Evento.valor"=w306) -> ()  [unwired: 9 in, 1 out]
                n168 = property on="Modo Propulsion" class="Bool (strict)"("BoolText.Text"="Activar Modo\n de Propulsón" ("Boolean Text.Text")) -> ()  [unwired: 2 in, 2 out]
              }
              frame True {
                n169 = call "Agregar evento al historial.vi"("Evento.nombre"="Modo Propulsión Activado", "Evento.valor"=w310) -> ()  [unwired: 9 in, 1 out]
                n170 = property on="Modo Propulsion" class="Bool (strict)"("BoolText.Text"="Desactivar Modo\nde Propulsión" ("Boolean Text.Text")) -> ()  [unwired: 2 in, 2 out]
              }
            }
            n171 = Merge Errors(w301) -> (w304:errorcluster)
            n172 = shared-variable-write(refnum<k21> "ni.var.psp://EmuGenV2/VariablesEmuGenV2/Modo Propulsion" ("shared variable refnum in"), w298) -> ()  [unwired: 1 in, 2 out]
          }
          frame "Abrir Ventana de Historial" {
            # "Mostrar ventana de historial"
            n173 = Variant To Data(type=refnum<vi> refnum ("Sub Panel"), Variant=w314) -> (data=w313:refnum<vi>, error out=w312:errorcluster)  [unwired: 1 in]
            n174 = call "Mostrar en SubPanel.vi"("error in (no error)"=w312, "Subpanel Ref"=w313) -> ("error out"=w311:errorcluster)  [unwired: 9 in]
            n175 = Merge Errors(w311, w318) -> (w317:errorcluster)
          }
          frame "Abrir Ventana de Pruebas" {
            # "Mostrar ventana de historial"
            n176 = Variant To Data(type=refnum<vi> refnum ("Sub Panel"), Variant=w322) -> (data=w321:refnum<vi>, error out=w320:errorcluster)  [unwired: 1 in]
            n177 = call "Mostrar en Subpanel.vi"("error in (no error)"=w320, "Subpanel Ref"=w321) -> ("error out"=w319:errorcluster)  [unwired: 9 in]
            n178 = Merge Errors(w319, w326) -> (w325:errorcluster)
          }
          frame "Abrir Ventana de Graficas" {
            # "Mostrar ventana de Gráficas"
            n179 = Variant To Data(error in=w328, type=refnum<vi> refnum ("Sub Panel"), Variant=w331) -> (data=w330:refnum<vi>, error out=w329:errorcluster)
            n180 = call "Mostrar en SubPanel.vi"("error in (no error)"=w329, "SubPnl Refnum"=w330) -> ("error out"=w327:errorcluster)  [unwired: 9 in]
          }
          frame "Abrir Ventana de Fallas" {
            # "Mostrar ventana de historial"
            n181 = Variant To Data(type=refnum<vi> refnum ("Sub Panel"), Variant=w338) -> (data=w336:refnum<vi>, error out=w334:errorcluster)  [unwired: 1 in]
            n182 = call "Mostrar en SubPanel.vi"("error in (no error)"=w334, "Subpanel Ref"=w336) -> ("error out"=w335:errorcluster)  [unwired: 9 in]
            n183 = Merge Errors(w335, w341) -> (w340:errorcluster)
          }
          frame "--- Exit and Error Handling---" {
            # "Separator - The following cases handle errors and exit messages."
            n184 = call-poly <vilib>:"Delacor_lib_QMH_Enqueue Message (poly).vi"("Priority Message? (F)"=TRUE, "Message Data"=T8 {"Origin"="", "Exit via Stop Module Req?"=FALSE, "Wait for Module to stop?"=FALSE} ("Stop Argument"), "Message"="Exit", "Message Queue in"=w346) -> ("error out"=w342:errorcluster)  [unwired: 6 in, 1 out]
          }
          frame "Simulate MHL Error" {
            # "#DQMH_HowTo The 'Simulate MHL Error' button  illustrates how the MHL handles errors. This event is instructional in nature and can be removed."
            # "Simulate an error occurring at the MHL"
            n185 = call "Module Name--constant.vi"() -> ("Module Name"=w348:string)  [unwired: 11 in]
            n186 = xnode "Error Ring"("parameter 0"=w348) -> ("error out"=w350:errorcluster)
            n187 = Merge Errors(w352, w350) -> (w351:errorcluster)
          }
          frame "Error" {
            # "#CodeRecommended - If you ever change the name of this \"Error\" message, you'll need to update the name in the Check Loop Error.vi as well."
            # "#CodeRecommended - If the module is running in standalone mode (External Launch = FALSE), this code will pop up an error dialog and call the 'Exit' message if an error occurs. Add more fine-grained error handling here."
            # "Error - Check the error message data and respond accordingly. This message is sent by the \"Error Handler\" VIs at the end of each loop in this application."
            n188 = property class="Module Admin"(reference=w362) -> ("Accessors:External Launch"=w361:bool)  [unwired: 1 in, 2 out]
            n189 = Variant To Data(error in=w370, type=errorcluster {"status"=FALSE, "code"=0, "source"=""} ("error constant"), Variant=w364) -> (data=w371:errorcluster, error out=w368:errorcluster)
            n190 = call "Module Name--constant.vi"() -> ("Module Name"=w360:string)  [unwired: 11 in]
            n191 = call "Error Reported.vi"("Additional Information"=w360, "Error"=w371) -> ()  [unwired: 9 in, 1 out]
            n192 = case shown="False" w361 {
              tunnel: [w376 _] -> w367
              tunnel: w363 -> [w374 _]
              tunnel: w371 -> [w375 _]
              frame False {
                # "If the module is running standalone, then pop up an error dialog and call the \"Exit\" message."
                n193 = call <vilib>:"Simple Error Handler.vi"("error in (no error)"=w375) -> ()  [unwired: 4 in, 5 out]
                n194 = call-poly <vilib>:"Delacor_lib_QMH_Enqueue Message (poly).vi"("Priority Message? (F)"=TRUE, "Message"="Exit", "Message Queue in"=w374) -> ("error out"=w376:errorcluster)  [unwired: 7 in, 1 out]
              }
              frame True {
                # "If the module was launched externally, calling the Error Reported broadcast VI is the only action performed by the \"Error\" message. The module's caller can then process the error appropriately."
              }
            }
            n195 = Merge Errors(w368, w367) -> (w366:errorcluster)
            n196 = local write "error out"(w366) -> ()
          }
          frame "Exit" {
            w381 = 91  # 91: not all Exit messages will have an argument
            w383 = TRUE  # Stop the VI
            # "Release the message queue reference"
            # "Exit - Exit the application."
            n197 = Variant To Data(error in=w391, type=T8 {"Origin"="", "Exit via Stop Module Req?"=FALSE, "Wait for Module to stop?"=FALSE} ("Stop Argument"), Variant=w382) -> (data=w379:T8, error out=w387:errorcluster)
            n198 = call <vilib>:"Clear Errors.vi"("error in (no error)"=w387, "specific error code to clear (0: all)"=w381) -> ("error out"=w390:errorcluster)  [unwired: 4 in, 1 out]
            n199 = control-ref of="This VI"() -> (w378:refnum<vi>)
            n200 = call "Handle Exit.vi"("Stop Argument"=w379, "Admin in"=w377, "VI reference"=w378) -> ("error out"=w386:errorcluster)  [unwired: 7 in, 1 out]
            n201 = call-dynamic "Delacor_lib_QMH_Release Message Queue.vi"("error in (no error)"=w390, "Message Queue"=w385) -> ("error out"=w389:errorcluster)  [unwired: 9 in]
            n202 = Merge Errors(w389, w386) -> (w388:errorcluster)
            n203 = call "Stop Module.vi"() -> ()  [unwired: 11 in, 1 out]
            n204 = call "Stop Module.vi"() -> ()  [unwired: 11 in, 1 out]
            n205 = call "Stop Module.vi"() -> ()  [unwired: 11 in, 1 out]
            n206 = call "Stop Module.vi"() -> ()  [unwired: 11 in, 1 out]
          }
          frame Default {
            # "'Default' case only runs if there is a message that isn't defined in any of the other cases.  Output a programming error."
            n207 = call "Module Name--constant.vi"() -> ("Module Name"=w392:string)  [unwired: 11 in]
            n208 = xnode "Error Ring"("parameter 0"=w393, "parameter 1"=w392) -> ("error out"=w397:errorcluster)
            n209 = Merge Errors(w395, w397) -> (w396:errorcluster)
          }
        }
        n210 = call-dynamic "Delacor_lib_QMH_Error Handler - Message Handling Loop.vi"("error in (no error)"=w199, "Message Queue in"=w189) -> ("dup error in"=w196:errorcluster)  [unwired: 8 in, 1 out]
      }
      n211 = while {
        tunnel: w33 -> [_]
        stop <- w47 stop-if-true
        n212 = Wait (ms)(milliseconds to wait=u32 100) -> ()  [unwired: 1 out]
        n213 = Get Date/Time In Seconds() -> (seconds since 1Jan1904=w50:timestamp)
        n214 = shared-variable-read(refnum<k21> "ni.var.psp://EmuGenV2/VariablesEmuGenV2/BUS DC ON" ("shared variable refnum in")) -> (→"Bus DC Encendido":bool)  [unwired: 1 in, 2 out]
        n215 = Format Date/Time String(time format string (%c)="%d/%m/%Y\n%I:%M:%S %p", seconds (now)=w50) -> (date/time string=→"date/time string":string)  [unwired: 1 in]
        n216 = local read "stop?"() -> (w47:bool)
      }
    }
    frame Error {
      # "Synchronize Caller Events.vi will inform Start Module.vi that the module has launched and will let the code calling Start Module.vi register for broadcasts and would permit the caller receive the broadcast that an error occurred at launch time."
      n217 = call-dynamic "Delacor_lib_QMH_Release Message Queue.vi"("error in (no error)"=w408, "Message Queue"=w406) -> ("error out"=w407:errorcluster)  [unwired: 9 in]
      n218 = call "Synchronize Caller Events.vi"("Singleton Module Admin in"=w409) -> ("error out"=w414:errorcluster)  [unwired: 9 in, 1 out]
      n219 = call "Module Name--constant.vi"() -> ("Module Name"=w412:string)  [unwired: 11 in]
      n220 = Format Into String(format string="An error occurred during initialization. %s is no longer running.", w412) -> (resulting string=w410:string)  [unwired: 2 in, 1 out]
      n221 = Merge Errors(w407, w414) -> (w415:errorcluster)
      n222 = call "Error Reported.vi"("Additional Information"=w410, "Error"=w415) -> ()  [unwired: 9 in, 1 out]
    }
  }
  n223 = Merge Errors(w29, w32) -> (w28:errorcluster)
  n224 = call "Close Module.vi"("error in (no error)"=w28, "Module Admin in"=w24) -> ("error out"=w30:errorcluster, "External Launch"=w18:bool, "Module Admin out"=w19:refnum<class "Delacor_lib_QMH_Module Admin.lvclass">)  [unwired: 7 in]
  n225 = Unregister For Events(event registration refnum=w23, error in=w30) -> (error out=w27:errorcluster)
  "error out" <- w27
  n226 = local write "Module Admin"(w19) -> ()
  n227 = case "External Launch?" shown="True" w18 {
    tunnel: w27 -> [_ w416]
    frame False {
    }
    frame True {
      n228 = case shown="Error" w416 {
        frame No Error {
          n229 = disable-structure shown="Disabled" {
            frame Disabled {
              n230 = invoke class="VI" method="FP.Close"() -> ()  [unwired: 3 in, 3 out]
            }
            frame Enabled {
            }
          }
        }
        frame Error {
          n231 = invoke class="VI" method="FP.Open"("Activate"=TRUE ("Activate?")) -> ()  [unwired: 4 in, 5 out]
        }
      }
    }
  }
